vi "RGBtoGreyscale.vi"(1 "RBG":u32[][](array[numeric])) -> (0 "Greyscale":u8[][](array[numeric]))   [LabVIEW 2020, in "g_ar_toolkit.test.lvlib" / "Image.lvclass"]
uses:
  Image.lvclass
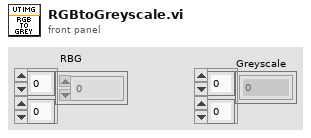
[diagram p1: front panel]
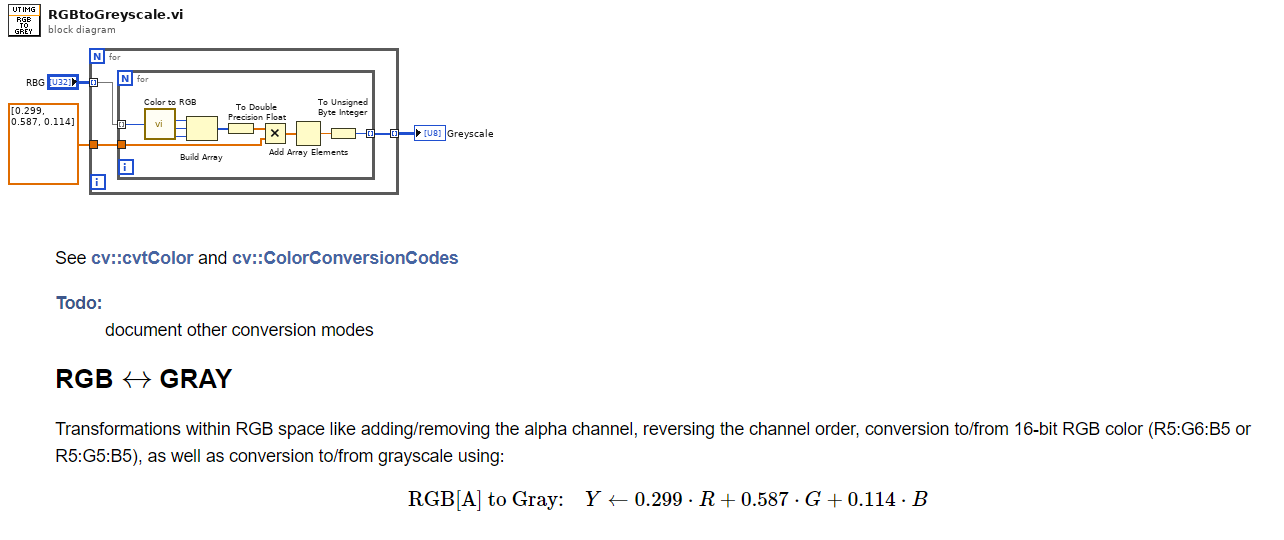
[diagram p0: block diagram]
diagram:
  n1 = for {
    tunnel: "RBG" -> [w6] mode=indexing
    tunnel: dbl[] [0.299, 0.587, 0.114] ("double precision float") -> [w5]
    tunnel: [w4] -> w1 mode=indexing
    n2 = for {
      tunnel: w6 -> [w10] mode=indexing
      tunnel: w5 -> [w11]
      tunnel: [w7] -> w4 mode=indexing
      n3 = call <vilib>:"Color to RGB.vi"("Color"=w10) -> ("R"=w16:u8, "G"=w15:u8, "B"=w14:u8)  [unwired: 1 out]
      n4 = Build Array(w16, w15, w14) -> (w13:u8[])
      n5 = To Double Precision Float(number=w13) -> (double precision float=w12:dbl[])
      n6 = Multiply(x=w12, y=w11) -> (x*y=w9:dbl[])
      n7 = Add Array Elements(numeric array=w9) -> (sum=w8:dbl)
      n8 = To Unsigned Byte Integer(number=w8) -> (unsigned 8bit integer=w7:u8)
    }
  }
  "Greyscale" <- w1
